vi "Stepper RT.vi"() -> ()   [LabVIEW 2012]
uses:
  <vilib>/FPGAPlugInAG/cRIO-9074/niLvFpga_Open_cRIO-9074.vi
  <vilib>/rvi/interface/common/dynamic/niFpgaDynamicAddResources.vi
  <vilib>/Utility/error.llb/Error Cluster From Error Code.vi
  <vilib>/rvi/errors/niLvFpgaAdjustHostInterfaceError.vi
  <vilib>/FPGAPlugInAG/Dynamic/niLvFpga_Close_Dynamic.vi
  <vilib>/rvi/interface/nirviOpenFPGA/nirviOpenFPGA.xnode
  FPGA Bitfiles/ActuationLabProj_FPGATarget_StepperFPGA_5A65D4EE.lvbitx
  Stepper FPGA.vi
  <vilib>/rvi/interface/nirviReadWriteControl/nirviReadWriteControl.xnode
  <vilib>/rvi/interface/nirviCloseFPGA/nirviCloseFPGA.xnode
  <vilib>/rvi/interface/Simulation/niFpgaSimulationCallBeginRW.vi
  NiFpgaLv.dll
panel:
  out "x >= y?":bool
  out "Heartbeat":bool
  in  "Stepper Motor Position (deg)":i32(knob) scale=0.0..359.0
  in  "stop":bool
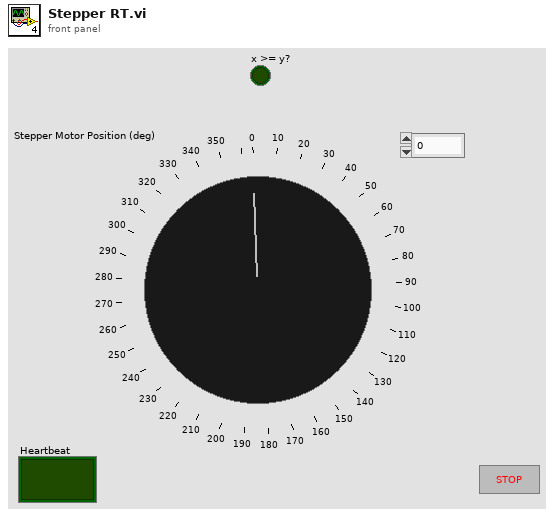
[diagram p1: front panel]
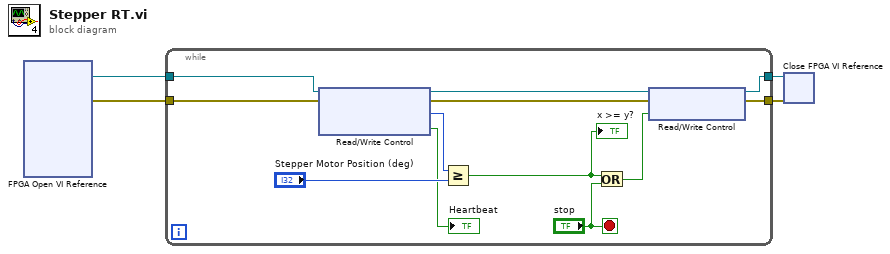
[diagram p0: block diagram]
diagram:
  n1 = xnode "FPGA Open VI Reference"() -> ("FPGA VI Reference Out"=w4:refnum<k20>, "error out"=w2:errorcluster)  [unwired: 2 in]
  n2 = while {
    tunnel: w4 -> [w16]
    tunnel: [w11] -> w3
    tunnel: w2 -> [w15]
    tunnel: [w9] -> w1
    stop <- "stop" stop-if-true
    n3 = xnode "Read/Write Control"("FPGA VI Reference In"=w16, "error in"=w15) -> ("FPGA VI Reference Out"=w12:refnum<k20>, "error out"=w10:errorcluster, "Absolute Position"=w14:i32, "Heartbeat"=→"Heartbeat":bool)
    n4 = Greater Or Equal?(x=w14, y="Stepper Motor Position (deg)") -> (x >= y?=w6:bool)
    "x >= y?" <- w6
    n5 = Or(x=w6, y="stop") -> (x .or. y?=w5:bool)
    n6 = xnode "Read/Write Control"("FPGA VI Reference In"=w12, "error in"=w10, "Enable/Disable"=w5) -> ("FPGA VI Reference Out"=w11:refnum<k20>, "error out"=w9:errorcluster)
  }
  n7 = xnode "Close FPGA VI Reference"("FPGA VI Reference In"=w3, "error in"=w1) -> ()  [unwired: 1 out]
